vi "Lucrarea 7.vi"() -> ()   [LabVIEW 2021]
panel:
  in  "Play Button":bool
  in  "Stop Button":bool
  out "Waveform Chart":dbl(graph)
  in  "A":dbl(slide)
  in  "k":dbl(slide)=0.5 min=0.5 max=10.0 step=0.5
  in  "m":dbl(slide)=0.5 min=0.5 max=10.0 step=0.5
  out "2D Picture":picture
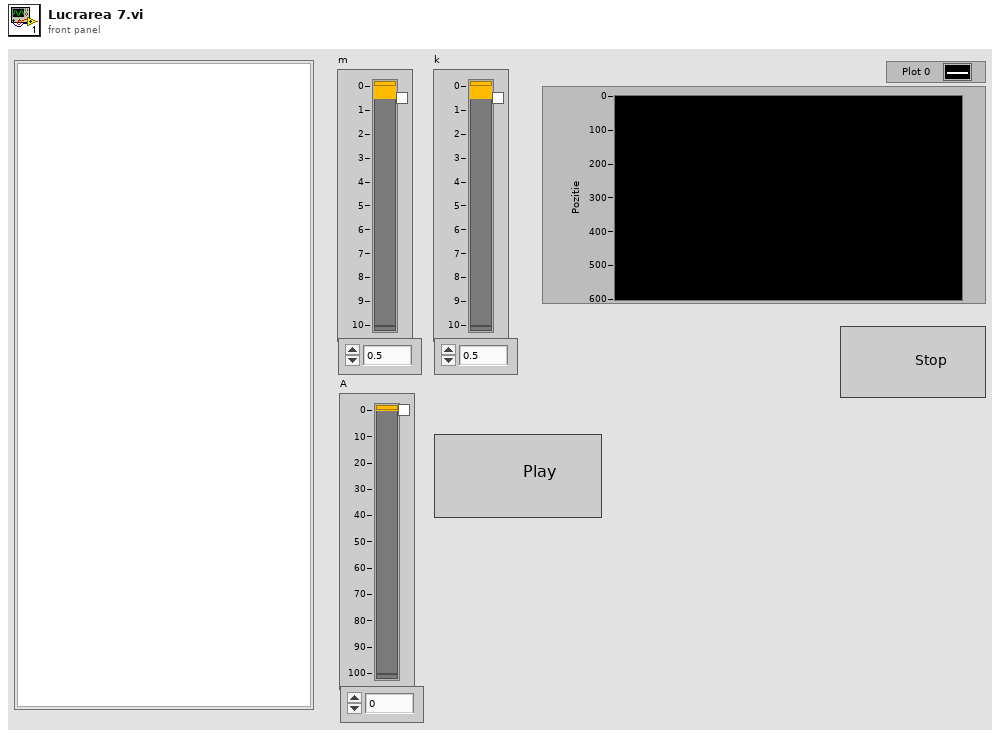
[diagram p1: front panel]
types:
  T1 = cluster{"Width":u16, "Style":enum32{"Solid", "Dash", "Dot", "DashDot", "DashDotDot"}}
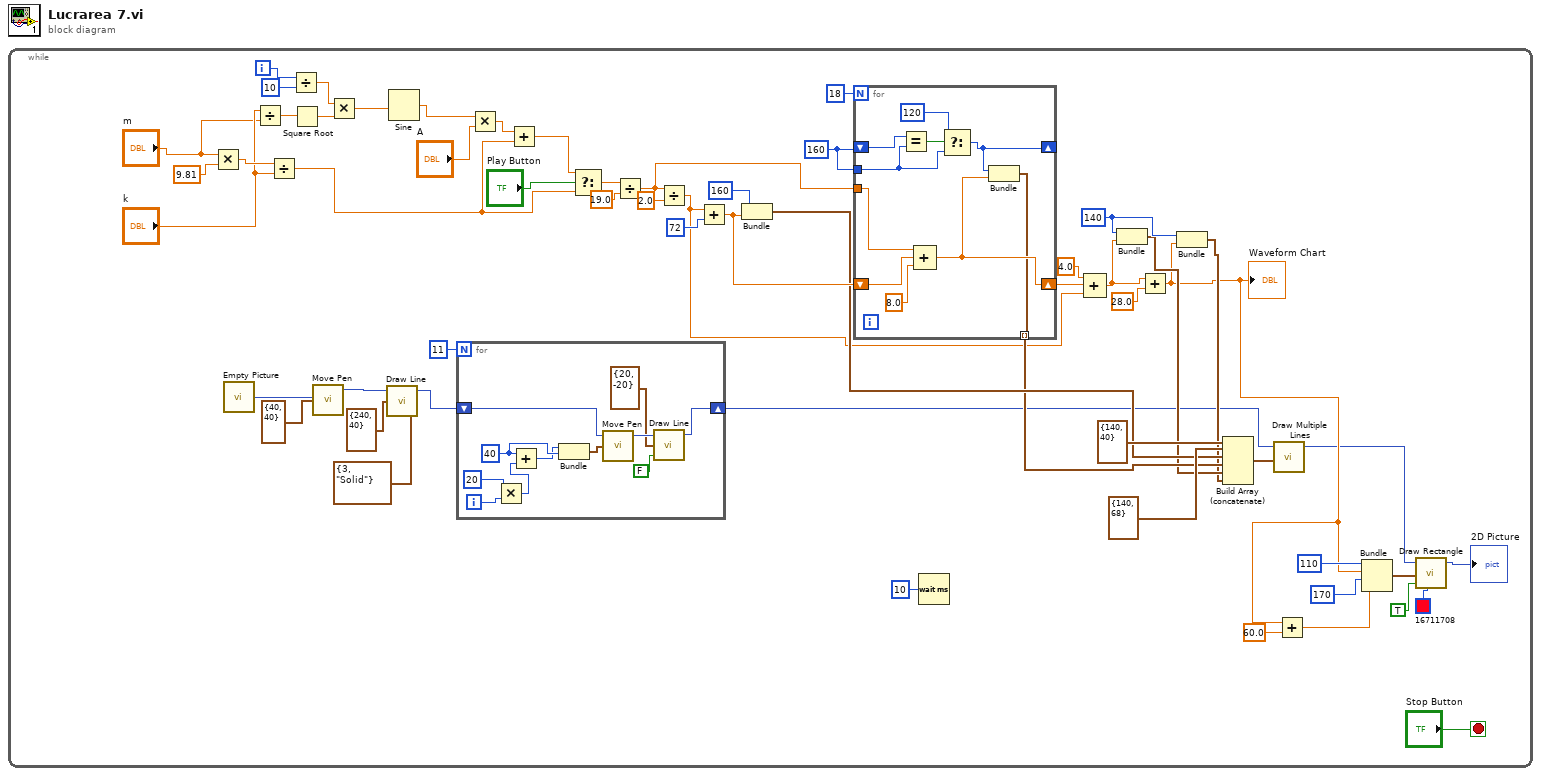
[diagram p0: block diagram]
diagram:
  n1 = while {
    i -> [w43]
    stop <- "Stop Button" stop-if-true
    w21 = 140 ("t")
    w28 = 160
    n2 = Multiply(x="m", y=9.81) -> (x*y=w50:dbl)
    n3 = call "Empty Picture"() -> ("empty picture"=w58:picture)
    n4 = Divide(x="k", y="m") -> (x/y=w47:dbl)
    n5 = Divide(x=w50, y="k") -> (x/y=w37:dbl)
    n6 = Divide(x=w43, y=10) -> (x/y=w45:dbl)
    n7 = Square Root(x=w47) -> (sqrt(x)=w46:dbl)
    n8 = call <vilib>:"Move Pen.vi"("new position"=cluster{"x":i16, "y":i16} {"x"=40, "y"=40}, "picture"=w58) -> ("new picture"=w56:picture)  [unwired: 3 in]
    n9 = Multiply(x=w45, y=w46) -> (x*y=w41:dbl)
    n10 = call <vilib>:"Draw Line.vi"("picture"=w56, "end point"=cluster{"x":i16, "y":i16} {"x"=240, "y"=40}, "pen"=T1 {"Width"=3, "Style"=enum."Solid"}) -> ("new picture"=w52:picture)  [unwired: 6 in]
    n11 = Sine(x=w41) -> (sin(x)=w40:dbl)
    n12 = for {
      N: 11 -> [_]
      shift-right: [w69] -> w13
      shift-left: w52 -> [w73]
      i -> [w78]
      w76 = 40 ("x")
      n13 = Multiply(x=20, y=w78) -> (x*y=w79:i32)
      n14 = Add(x=w76, y=w79) -> (x+y=w75:i32)
      n15 = Bundle(w75, "x"=w76) -> (w74:cluster{i32, "x":i32})  [unwired: 1 in]
      n16 = call <vilib>:"Move Pen.vi"("new position"=w74, "picture"=w73) -> ("new picture"=w72:picture)  [unwired: 3 in]
      n17 = call <vilib>:"Draw Line.vi"("picture"=w72, "end point"=cluster{"x":i16, "y":i16} {"x"=20, "y"=-20}, "absolute coordinates?(T)"=FALSE) -> ("new picture"=w69:picture)  [unwired: 6 in]
    }
    n18 = Multiply(x=w40, y="A") -> (x*y=w38:dbl)
    n19 = Add(x=w38, y=w37) -> (x+y=w35:dbl)
    n20 = Select(t=w35, s="Play Button", f=w37) -> (s? t:f=w34:dbl)
    n21 = Divide(x=w34, y=19.0) -> (x/y=w27:dbl)
    n22 = Divide(x=w27, y=2.0) -> (x/y=w2:dbl)
    n23 = Add(x=w2, y=72) -> (x+y=w26:dbl)
    n24 = Bundle(160, w26) -> (w18:cluster{i32, dbl})  [unwired: 1 in]
    n25 = for {
      N: 18 -> [_]
      shift-right: [w61] -> _
      shift-left: w28 -> [w64]
      tunnel: w28 -> [w63]
      tunnel: w27 -> [w68]
      shift-right: [w60] -> w25
      shift-left: w26 -> [w67]
      tunnel: [w59] -> w17 mode=indexing
      n26 = Equal?(x=w64, y=w63) -> (x = y?=w65:bool)
      n27 = Compound Arithmetic op=ADD(w68, w67, 8.0 ("value")) -> (w60:dbl)
      n28 = Select(t=120, s=w65, f=w63) -> (s? t:f=w61:i32)
      n29 = Bundle("t"=w61, w60) -> (w59:cluster{"t":i32, dbl})  [unwired: 1 in]
    }
    n30 = Wait (ms)(milliseconds to wait=u32 10) -> ()  [unwired: 1 out]
    n31 = Compound Arithmetic op=ADD(4.0 ("value"), w25, w2) -> (w23:dbl)
    n32 = Bundle("t"=w21, w23) -> (w16:cluster{"t":i32, dbl})  [unwired: 1 in]
    n33 = Add(x=w23, y=28.0) -> (x+y=w10:dbl)
    "Waveform Chart" <- w10
    n34 = Bundle("t"=w21, w10) -> (w15:cluster{"t":i32, dbl})  [unwired: 1 in]
    n35 = Build Array (concatenate)(cluster{"x":i16, "y":i16} {"x"=140, "y"=40} ("end point"), cluster{"x":i16, "y":i16} {"x"=140, "y"=68} ("end point"), w18, w17, w16, w15) -> (w14:cluster{"t":i32, "y":dbl}[])
    n36 = call <vilib>:"Draw Multiple Lines.vi"("picture"=w13, "line endpoints"=w14) -> ("new picture"=w3:picture)  [unwired: 7 in]
    n37 = Add(x=w10, y=60.0) -> (x+y=w8:dbl)
    n38 = Bundle("x"=i16 110, w10, "x"=i16 170, w8) -> (w6:cluster{"x":i16, dbl, "x":i16, dbl})  [unwired: 1 in]
    n39 = call <vilib>:"Draw Rectangle.vi"("picture"=w3, "rect"=w6, "fill?(F)"=TRUE, "color(black)"=u32 16711708) -> ("new picture"=→"2D Picture":picture)  [unwired: 5 in]
  }
